vi "Example Test 4.vi"() -> ()   [LabVIEW 2018]
panel:
  out "array out":string[](array[string])
  out "Error Out":errorcluster
  in  "Error In":errorcluster
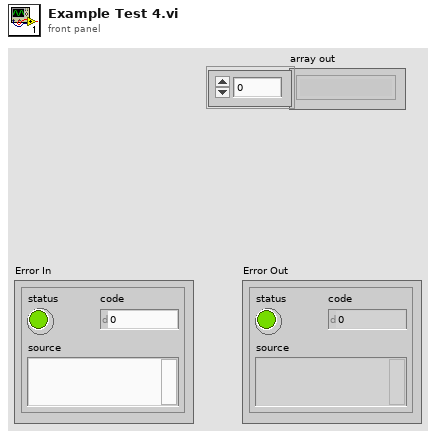
[diagram p1: front panel]
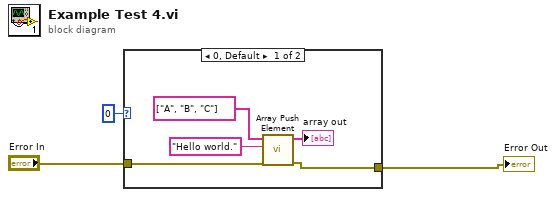
[diagram p0: block diagram]
diagram:
  n1 = case shown="0, Default" 0 {
    tunnel: [w7 w9] -> w3
    tunnel: "Error In" -> [w8 w9]
    frame 0, Default {
      n2 = call "Array Push Element.vi"("Error In"=w8, "element"="Hello world.", "array in"=string[] ["A", "B", "C"]) -> ("Error Out"=w7:errorcluster, "array out"=→"array out":string[])  [unwired: 7 in]
    }
    frame 1 {
    }
  }
  "Error Out" <- w3
